vi "RP get info.vi"(5 "Ranges":dbl[](array[numeric])=[20.0, 1.0], 7 "Trigger offset":i32 format="0x%x (%d)", 8 "Error In":errorcluster, 9 "Channel names":string[](array[string])=["CH0", "CH1"], 10 "Delayed start":u64=571428 format="0x%x (%d)", 11 "connection ID":refnum<k5>) -> (0 "Error Out":errorcluster, 2 "Channel info":T1[](array[typedef]) {"waveform start" format="%#_6p"; "waveform period" format="%#_6p"}, 3 "connection ID out":refnum<k5>)   [LabVIEW 2015]
uses:
  RP info.ctl
  RP Config Offsets.ctl
  RP Status Offsets.ctl
panel:
  out "Status response 2":u32=1 format="0x%x (%d)"
  out "Status response":u32=1 format="0x%x (%d)"
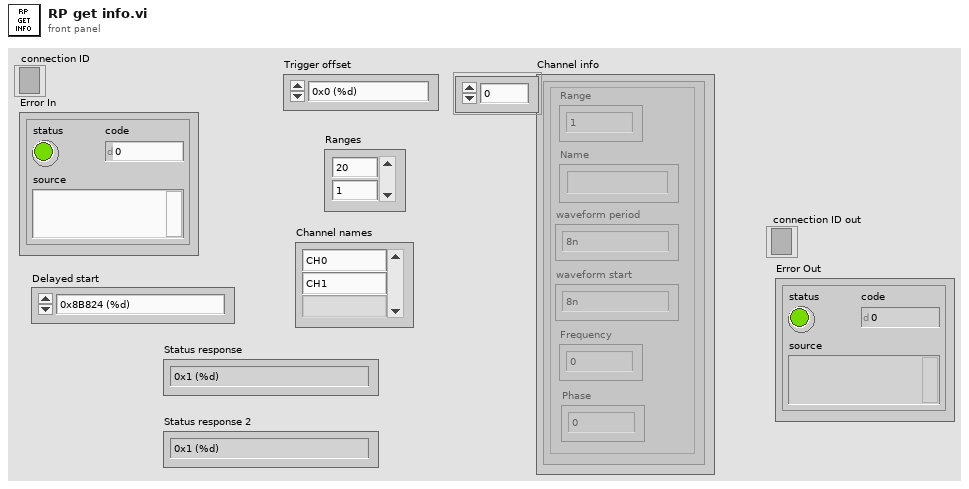
[diagram p1: front panel]
types:
  T1 = typedef "RP info.ctl" = cluster{"Range":dbl, "Name":string, "waveform period":dbl, "waveform start":dbl, "Frequency":u32, "Phase":u32}
  T2 = typedef "RP Status Offsets.ctl" = u16
  T3 = typedef "RP Config Offsets.ctl" = u16
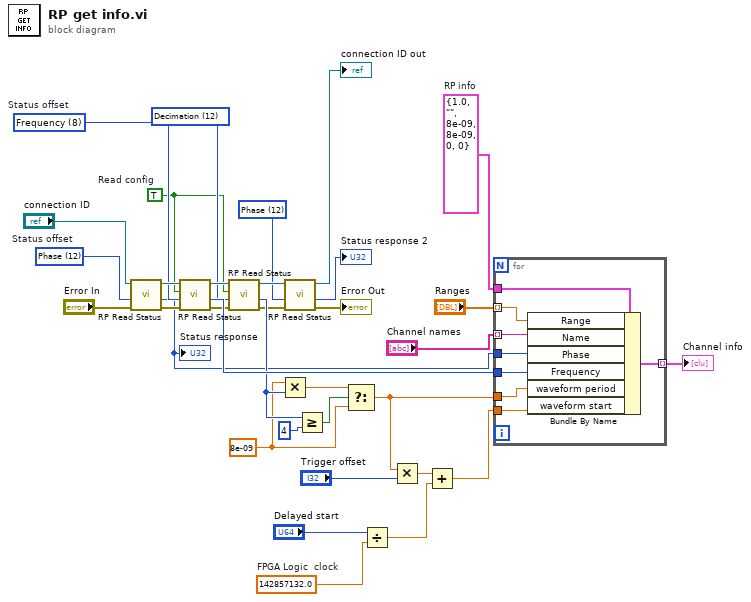
[diagram p0: block diagram]
diagram:
  w4 = 142857132.0  # FPGA Logic  clock
  w7 = T2 12 items=["Writer address"=0, "Record start position"=4, "Trig state etc."=8, "Phase"=12, "RxFIFO counter"=24, "TxFIFO counter"=28] ("Status offset")
  w15 = 8e-09
  w22 = T3 12 items=["Config flags"=0, "Record length"=4, "Frequency"=8, "Decimation"=12, "LED"=16, "DDS delay"=28] ("Status offset")
  w26 = T3 8 items=["Config flags"=0, "Record length"=4, "Frequency"=8, "Decimation"=12, "LED"=16, "DDS delay"=28]  # Status offset
  w21 = TRUE  # Read config
  w31 = T1 {"Range"=1.0, "Name"="", "waveform period"=8e-09, "waveform start"=8e-09, "Frequency"=0, "Phase"=0}  # RP info
  w32 = T2 12 items=["Writer address"=0, "Record start position"=4, "Trig state etc."=8, "Phase"=12, "RxFIFO counter"=24, "TxFIFO counter"=28]  # Status offset
  n1 = call "RP Read Status.vi"("Error In"="Error In", "Status offset"=w32, "connection ID"="connection ID") -> ("Error Out"=w25:errorcluster, "Status response"=w12:u32, "connection ID out"=w27:refnum<k5>)  [unwired: 6 in]
  "Status response" <- w12
  n2 = call "RP Read Status.vi"("Error In"=w25, "Status offset"=w26, "Read config"=w21, "connection ID"=w27) -> ("Error Out"=w20:errorcluster, "Status response"=w24:u32, "connection ID out"=w23:refnum<k5>)  [unwired: 5 in]
  n3 = call "RP Read Status.vi"("Error In"=w20, "Status offset"=w22, "Read config"=w21, "connection ID"=w23) -> ("Error Out"=w10:errorcluster, "Status response"=w18:u32, "connection ID out"=w9:refnum<k5>)  [unwired: 5 in]
  n4 = Multiply(x=w15, y=w18) -> (x*y=w17:dbl)
  n5 = call "RP Read Status.vi"("Error In"=w10, "Status offset"=w7, "connection ID"=w9) -> ("Error Out"=→"Error Out":errorcluster, "Status response"=→"Status response 2":u32, "connection ID out"=→"connection ID out":refnum<k5>)  [unwired: 6 in]
  n6 = Greater Or Equal?(x=w18, y=u32 4) -> (x >= y?=w16:bool)
  n7 = Select(t=w17, s=w16, f=w15) -> (s? t:f=w13:dbl)
  n8 = Divide(x="Delayed start", y=w4) -> (x/y=w1:dbl)
  n9 = Multiply(x=w13, y="Trigger offset") -> (x*y=w2:dbl)
  n10 = Add(x=w2, y=w1) -> (x+y=w3:dbl)
  n11 = for {
    tunnel: w31 -> [w42]
    tunnel: "Ranges" -> [w41] mode=indexing
    tunnel: "Channel names" -> [w40] mode=indexing
    tunnel: [w39] -> w28 mode=indexing
    tunnel: w12 -> [w38]
    tunnel: w24 -> [w37]
    tunnel: w13 -> [w36]
    tunnel: w3 -> [w35]
    n12 = Bundle By Name(cluster=w42, "Range"=w41, "Name"=w40, "Phase"=w38, "Frequency"=w37, "waveform period"=w36, "waveform start"=w35) -> (w39:T1)
  }
  "Channel info" <- w28
